vi "UserInterface.vi"() -> ()   [LabVIEW 2017]
uses:
  <vilib>/Instr/_visa.llb/VISA Configure Serial Port (Instr).vi
  <vilib>/Utility/inputDevices.llb/joystickAcquire.vi
panel:
  out "Y-Axis":string
  out "joystick info":T1(array[cluster])
  out "Xbee: Data Received":string
  in  "Read":bool
  in  "Write":bool
  in  "Stop":bool
  out "axis info":T2
  out "X-Axis":string
  in  "XBEE-1":refnum<visa-resource-name>
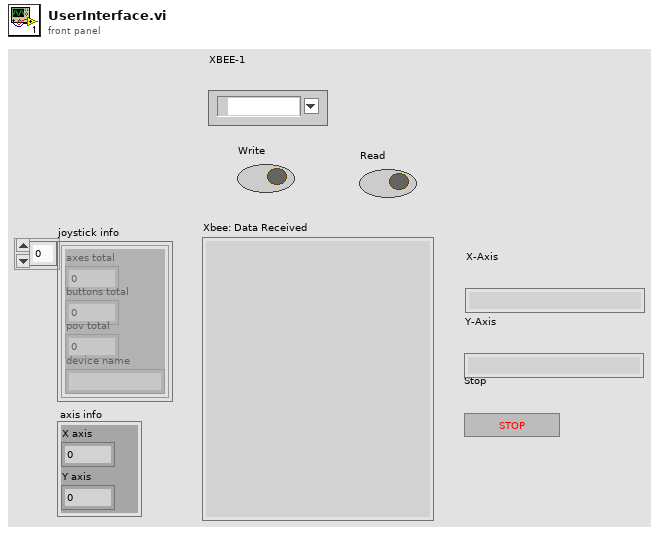
[diagram p1: front panel]
types:
  T1 = cluster{"axes total":u32, "buttons total":u32, "pov total":u32, "device name":string}[]
  T2 = cluster{"X axis":i32, "Y axis":i32, "Z axis":i32, "X axis rotation":i32, "Y axis rotation":i32, "Z axis rotation":i32, "U axis":i32, "V axis":i32}
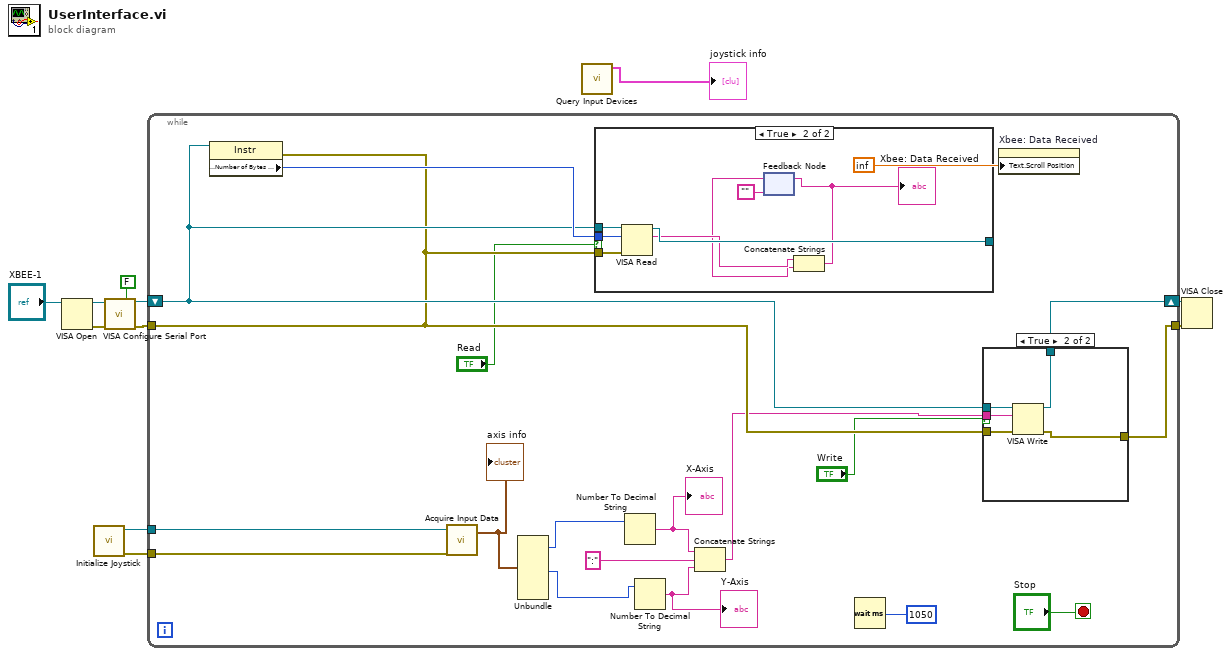
[diagram p0: block diagram]
diagram:
  n1 = VISA Open(VISA resource name="XBEE-1") -> (VISA resource name=w6:refnum<visa-resource-name>, error out=w5:errorcluster)  [unwired: 4 in]
  n2 = call <vilib>:"Initialize Joystick.vi"() -> ("error out"=w7:errorcluster, "device ID"=w8:refnum<k1>)  [unwired: 10 in]
  n3 = call-poly "VISA Configure Serial Port"("VISA resource name"=w6, "Enable Termination\nChar (T)"=FALSE ("Enable Termination\nChar (T)"), "error in (no error)"=w5) -> ("VISA resource name out"=w10:refnum<visa-resource-name>, "error out"=w9:errorcluster)  [unwired: 11 in]
  n4 = while {
    tunnel: [w22] -> w3
    tunnel: w9 -> [w24]
    tunnel: w8 -> [w26]
    tunnel: w7 -> [w27]
    shift-right: [w23] -> w2
    shift-left: w10 -> [w25]
    stop <- "Stop" stop-if-true
    n5 = property class="Instr"(reference=w25, error in=w24) -> ("Serial Settings:Number of Bytes at Serial Port"=w29:u32)  [unwired: 2 out]
    n6 = call-poly <vilib>:"Acquire Input Data.vi"("device ID"=w26, "error in (no error)"=w27) -> ("axis info"=w18:T2)  [unwired: 13 in, 4 out]
    "axis info" <- w18
    n7 = Unbundle(w18) -> ("Y axis"=w13:i32, "Y axis rotation"=w15:i32)  [unwired: 6 out]
    n8 = case shown="True" "Read" {
      tunnel: w29 -> [_ w46]
      tunnel: w25 -> [w38 w45]
      tunnel: w24 -> [_ w44]
      tunnel: [w38 w43] -> _
      frame False {
      }
      frame True {
        n9 = VISA Read(VISA resource name=w45, byte count=w46, error in (no error)=w44) -> (VISA resource name out=w43:refnum<visa-resource-name>, read buffer=w42:string)  [unwired: 2 out]
        n10 = feedback #1("") -> (w39:string)
        n11 = Concatenate Strings(w42, w39) -> (w40:string)
        "Xbee: Data Received" <- w40
        n12 = feedback-in #1(w40) -> ()
      }
    }
    n13 = Number To Decimal String(number=w13) -> (decimal integer string=w12:string)  [unwired: 1 in]
    "X-Axis" <- w12
    n14 = Number To Decimal String(number=w15) -> (decimal integer string=w14:string)  [unwired: 1 in]
    "Y-Axis" <- w14
    n15 = Concatenate Strings(w12, ":", w14) -> (w16:string)
    n16 = Wait (ms)(milliseconds to wait=u32 1050) -> ()  [unwired: 1 out]
    n17 = case shown="True" "Write" {
      tunnel: w25 -> [w32 w37]
      tunnel: w24 -> [w31 w36]
      tunnel: [w32 w35] -> w23
      tunnel: [w31 w34] -> w22
      tunnel: w16 -> [_ w33]
      frame False {
      }
      frame True {
        n18 = VISA Write(VISA resource name=w37, write buffer=w33, error in (no error)=w36) -> (VISA resource name out=w35:refnum<visa-resource-name>, error out=w34:errorcluster)  [unwired: 1 out]
      }
    }
    n19 = property on="Xbee: Data Received" class="Str"("Text.Scroll Position"=inf) -> ()  [unwired: 2 in, 2 out]
  }
  n20 = call <vilib>:"Query Input Devices.vi"() -> ("joystick info"=→"joystick info":T1)  [unwired: 8 in, 3 out]
  n21 = VISA Close(VISA resource name=w2, error in (no error)=w3) -> ()  [unwired: 1 out]
